vi "UI_(05A)_Set_Record_Start_State.vi"(3 "error in (no error)":errorcluster, 4 "Settings cluster in":T1={"Defaults"={"Default User"=0.0, "VISA Resource Name "="", "Histogram parameters"={"max"=300.0, "min"=0.0, "# bins"=10, "threshold"=8.0, "thr. type"=enum."higher accepted"}}, "Recording and saving"={"Researcher name"="", "Name prefix"="", "Data post-processing"={"Filter type"=enum."Savitzky-Golay", "Length"=31, "Order"=3}, "Stop at"=0.0, "\"Stop at\" enabled"=FALSE, "Default save folder path"=path "", "Acquisition FPS"=enum."Max"}, "Geometry"={"Sensor board size"=enum."", "Bridge swap"=FALSE, "Twisted neck"=FALSE, "Bridge H. offset"=0.0, "Bridge V. offset"=0.0, "Magnets orientation"=0.0, "Cage type"=0, "Cage parameters"={"Round"=variant(i16 0), "Square"=variant(u16 0), "Donut-maze"=variant(u16 0), "T-maze"=variant(u8 0), "Sociability-maze"=variant(u8 0)}}, "IO parameters"={"IO general config."=0, "IO 1 configuration"=0, "IO 2 configuration"=0, "IO 3 configuration"=0, "IO 4 configuration"=0, "Activate ext. RS-232"=0, "IO inversion config."=0, "Sync capability"=1}, "Conditions presets array"=[{"Enabled"=FALSE, "Name"="", "Specifier(s)"=[], "Response"={"Response type"=enum."Air puff", "TTL port"=enum."Port 1", "TTL pulse length, ms"=0.0}, "Has been set"=FALSE}, {"Enabled"=FALSE, "Name"="", "Specifier(s)"=[], "Response"={"Response type"=enum."Air puff", "TTL port"=enum."Port 1", "TTL pulse length, ms"=0.0}, "Has been set"=FALSE}, {"Enabled"=FALSE, "Name"="", "Specifier(s)"=[], "Response"={"Response type"=enum."Air puff", "TTL port"=enum."Port 1", "TTL pulse length, ms"=0.0}, "Has been set"=FALSE}, {"Enabled"=FALSE, "Name"="", "Specifier(s)"=[], "Response"={"Response type"=enum."Air puff", "TTL port"=enum."Port 1", "TTL pulse length, ms"=0.0}, "Has been set"=FALSE}, {"Enabled"=FALSE, "Name"="", "Specifier(s)"=[], "Response"={"Response type"=enum."Air puff", "TTL port"=enum."Port 1", "TTL pulse length, ms"=0.0}, "Has been set"=FALSE}, {"Enabled"=FALSE, "Name"="", "Specifier(s)"=[], "Response"={"Response type"=enum."Air puff", "TTL port"=enum."Port 1", "TTL pulse length, ms"=0.0}, "Has been set"=FALSE}, {"Enabled"=FALSE, "Name"="", "Specifier(s)"=[], "Response"={"Response type"=enum."Air puff", "TTL port"=enum."Port 1", "TTL pulse length, ms"=0.0}, "Has been set"=FALSE}, {"Enabled"=FALSE, "Name"="", "Specifier(s)"=[], "Response"={"Response type"=enum."Air puff", "TTL port"=enum."Port 1", "TTL pulse length, ms"=0.0}, "Has been set"=FALSE}, {"Enabled"=FALSE, "Name"="", "Specifier(s)"=[], "Response"={"Response type"=enum."Air puff", "TTL port"=enum."Port 1", "TTL pulse length, ms"=0.0}, "Has been set"=FALSE}, {"Enabled"=FALSE, "Name"="", "Specifier(s)"=[], "Response"={"Response type"=enum."Air puff", "TTL port"=enum."Port 1", "TTL pulse length, ms"=0.0}, "Has been set"=FALSE}, {"Enabled"=FALSE, "Name"="", "Specifier(s)"=[], "Response"={"Response type"=enum."Air puff", "TTL port"=enum."Port 1", "TTL pulse length, ms"=0.0}, "Has been set"=FALSE}, {"Enabled"=FALSE, "Name"="", "Specifier(s)"=[], "Response"={"Response type"=enum."Air puff", "TTL port"=enum."Port 1", "TTL pulse length, ms"=0.0}, "Has been set"=FALSE}, {"Enabled"=FALSE, "Name"="", "Specifier(s)"=[], "Response"={"Response type"=enum."Air puff", "TTL port"=enum."Port 1", "TTL pulse length, ms"=0.0}, "Has been set"=FALSE}, {"Enabled"=FALSE, "Name"="", "Specifier(s)"=[], "Response"={"Response type"=enum."Air puff", "TTL port"=enum."Port 1", "TTL pulse length, ms"=0.0}, "Has been set"=FALSE}], "Calibration parameters"={"Timing calibration sw/hw"=1.0, "True FPS"=80.0, "True frame time, s"=80.0, "Disp. calibration info"=[]}, "Settings loaded OK"=FALSE} {"Calibration parameters"."True frame time, s" format="%.10g"; "Calibration parameters"."Disp. calibration info"."Speed, µl per ms" format="%.3g"; "Calibration parameters"."True FPS" format="%.10g"; "Calibration parameters"."Timing calibration sw/hw" format="%.10g"; "Conditions presets array"."Specifier(s)"."Validity criteria(s)"."Validity value" min=0.0 step=0.1 format="%.2g"; "Conditions presets array"."Specifier(s)"."Value" step=1.0 format="%#.2g"; "Recording and saving"."Data post-processing"."Order" min=3 max=11 step=2; "Recording and saving"."Data post-processing"."Length" min=5 max=301 step=2; "Geometry"."Cage type" items=["Round", "Square", "Donut-maze", "T-maze", "Sociability maze", ""]}, 5 "All references in":T21) -> (0 "error out":errorcluster, 1 "Settings cluster out":T1={"Defaults"={"Default User"=0.0, "VISA Resource Name "="", "Histogram parameters"={"max"=300.0, "min"=0.0, "# bins"=10, "threshold"=8.0, "thr. type"=enum."higher accepted"}}, "Recording and saving"={"Researcher name"="", "Name prefix"="", "Data post-processing"={"Filter type"=enum."Savitzky-Golay", "Length"=31, "Order"=3}, "Stop at"=0.0, "\"Stop at\" enabled"=FALSE, "Default save folder path"=path "", "Acquisition FPS"=enum."Max"}, "Geometry"={"Sensor board size"=enum."", "Bridge swap"=FALSE, "Twisted neck"=FALSE, "Bridge H. offset"=0.0, "Bridge V. offset"=0.0, "Magnets orientation"=0.0, "Cage type"=0, "Cage parameters"={"Round"=variant(i16 0), "Square"=variant(u16 0), "Donut-maze"=variant(u16 0), "T-maze"=variant(u8 0), "Sociability-maze"=variant(u8 0)}}, "IO parameters"={"IO general config."=0, "IO 1 configuration"=0, "IO 2 configuration"=0, "IO 3 configuration"=0, "IO 4 configuration"=0, "Activate ext. RS-232"=0, "IO inversion config."=0, "Sync capability"=1}, "Conditions presets array"=[{"Enabled"=FALSE, "Name"="", "Specifier(s)"=[], "Response"={"Response type"=enum."Air puff", "TTL port"=enum."Port 1", "TTL pulse length, ms"=0.0}, "Has been set"=FALSE}, {"Enabled"=FALSE, "Name"="", "Specifier(s)"=[], "Response"={"Response type"=enum."Air puff", "TTL port"=enum."Port 1", "TTL pulse length, ms"=0.0}, "Has been set"=FALSE}, {"Enabled"=FALSE, "Name"="", "Specifier(s)"=[], "Response"={"Response type"=enum."Air puff", "TTL port"=enum."Port 1", "TTL pulse length, ms"=0.0}, "Has been set"=FALSE}, {"Enabled"=FALSE, "Name"="", "Specifier(s)"=[], "Response"={"Response type"=enum."Air puff", "TTL port"=enum."Port 1", "TTL pulse length, ms"=0.0}, "Has been set"=FALSE}, {"Enabled"=FALSE, "Name"="", "Specifier(s)"=[], "Response"={"Response type"=enum."Air puff", "TTL port"=enum."Port 1", "TTL pulse length, ms"=0.0}, "Has been set"=FALSE}, {"Enabled"=FALSE, "Name"="", "Specifier(s)"=[], "Response"={"Response type"=enum."Air puff", "TTL port"=enum."Port 1", "TTL pulse length, ms"=0.0}, "Has been set"=FALSE}, {"Enabled"=FALSE, "Name"="", "Specifier(s)"=[], "Response"={"Response type"=enum."Air puff", "TTL port"=enum."Port 1", "TTL pulse length, ms"=0.0}, "Has been set"=FALSE}, {"Enabled"=FALSE, "Name"="", "Specifier(s)"=[], "Response"={"Response type"=enum."Air puff", "TTL port"=enum."Port 1", "TTL pulse length, ms"=0.0}, "Has been set"=FALSE}, {"Enabled"=FALSE, "Name"="", "Specifier(s)"=[], "Response"={"Response type"=enum."Air puff", "TTL port"=enum."Port 1", "TTL pulse length, ms"=0.0}, "Has been set"=FALSE}, {"Enabled"=FALSE, "Name"="", "Specifier(s)"=[], "Response"={"Response type"=enum."Air puff", "TTL port"=enum."Port 1", "TTL pulse length, ms"=0.0}, "Has been set"=FALSE}, {"Enabled"=FALSE, "Name"="", "Specifier(s)"=[], "Response"={"Response type"=enum."Air puff", "TTL port"=enum."Port 1", "TTL pulse length, ms"=0.0}, "Has been set"=FALSE}, {"Enabled"=FALSE, "Name"="", "Specifier(s)"=[], "Response"={"Response type"=enum."Air puff", "TTL port"=enum."Port 1", "TTL pulse length, ms"=0.0}, "Has been set"=FALSE}, {"Enabled"=FALSE, "Name"="", "Specifier(s)"=[], "Response"={"Response type"=enum."Air puff", "TTL port"=enum."Port 1", "TTL pulse length, ms"=0.0}, "Has been set"=FALSE}, {"Enabled"=FALSE, "Name"="", "Specifier(s)"=[], "Response"={"Response type"=enum."Air puff", "TTL port"=enum."Port 1", "TTL pulse length, ms"=0.0}, "Has been set"=FALSE}], "Calibration parameters"={"Timing calibration sw/hw"=1.0, "True FPS"=80.0, "True frame time, s"=80.0, "Disp. calibration info"=[]}, "Settings loaded OK"=FALSE} {"Calibration parameters"."True frame time, s" format="%.10g"; "Calibration parameters"."Disp. calibration info"."Speed, µl per ms" format="%.3g"; "Calibration parameters"."True FPS" format="%.10g"; "Calibration parameters"."Timing calibration sw/hw" format="%.10g"; "Conditions presets array"."Specifier(s)"."Validity criteria(s)"."Validity value" min=0.0 step=0.1 format="%.2g"; "Conditions presets array"."Specifier(s)"."Value" step=1.0 format="%#.2g"; "Recording and saving"."Data post-processing"."Order" min=3 max=11 step=2; "Recording and saving"."Data post-processing"."Length" min=5 max=301 step=2; "Geometry"."Cage type" items=["Round", "Square", "Donut-maze", "T-maze", "Sociability maze", ""]}, 2 "All references out":T21)   [LabVIEW 2018, in "Tracker.lvlib"]
uses:
  Tracker.lvlib
  Controls/CTL_All_References.ctl
  Controls/CTL_Controls_References.ctl
  Controls/CTL_Indicators_References.ctl
  Controls/CTL_Panes_and_VIs_References.ctl
  Controls/CTL_Histogram_Properties.ctl
  <vilib>/Utility/miscctls.llb/LVRangeTypeDef.ctl
  Controls/CTL_Settings_cluster.ctl
  Controls/CTL_Histogram_parameters.ctl
  Controls/CTL_Filter_selector.ctl
  Controls/CTL_Acquisition_speed_selector.ctl
  Controls/CTL_Segmented_plot_parameters_2.ctl
  Libraries/Cage Diagram/Typedefs/CTL_Cage_type.ctl
  Controls/CTL_Cage_all_segmentation_params_set.ctl
  Controls/CTL_IO_params_cluster.ctl
  Controls/CTL_Conditions_Array.ctl
  Controls/CTL_Conditions_Cluster.ctl
  Controls/CTL_Condition_type.ctl
  Controls/CTL_Comparison_type.ctl
  Controls/CTL_Validity_check_criteria.ctl
  Controls/CTL_Response_info.ctl
  Controls/CTL_Condition_response_type.ctl
  Controls/CTL_Reponse_port_info.ctl
  Controls/CTL_Calibration_parameters.ctl
  Controls/CTL_Dispenser_calibration_info.ctl
  <vilib>/Utility/error.llb/Error Cluster From Error Code.vi
  <vilib>/ErrorRing/Error Ring.xnode
  Common_Resources.lvlib
  Libraries/Cage Diagram/Cage Diagram.lvlib
panel:
  in  "Histogram initialization cluster":T19={"X Scale.Range"={"Minimum"=0.0, "Maximum"=13.0, "Increment"=1.0, "Minor Increment"=1.0, "Start"=0.0}, "Caption.Text"="Zone preference (normalized)", "X Scale.Offset and Multiplier:Multiplier"=1.0, "X Scale.Offset and Multiplier:Offset"=0.0, "X Scale.Scale Fit"=2, "X Scale.Display Format:Precision"=0, "Y Scale.Mapping Mode"=0, "Zones preference empty initialized array"=[0, 0, 0, 0, 0, 0, 0, 0, 0, 0, 0, 0, 0, 0], "Plot.Fill/Point Color"=15790320}
  out "Panes references":T24
  out "Controls references params":string[][](array[string])
  out "Indicators references params":string[][](array[string])
  out "Indicators references":T23
  out "Controls references":T22
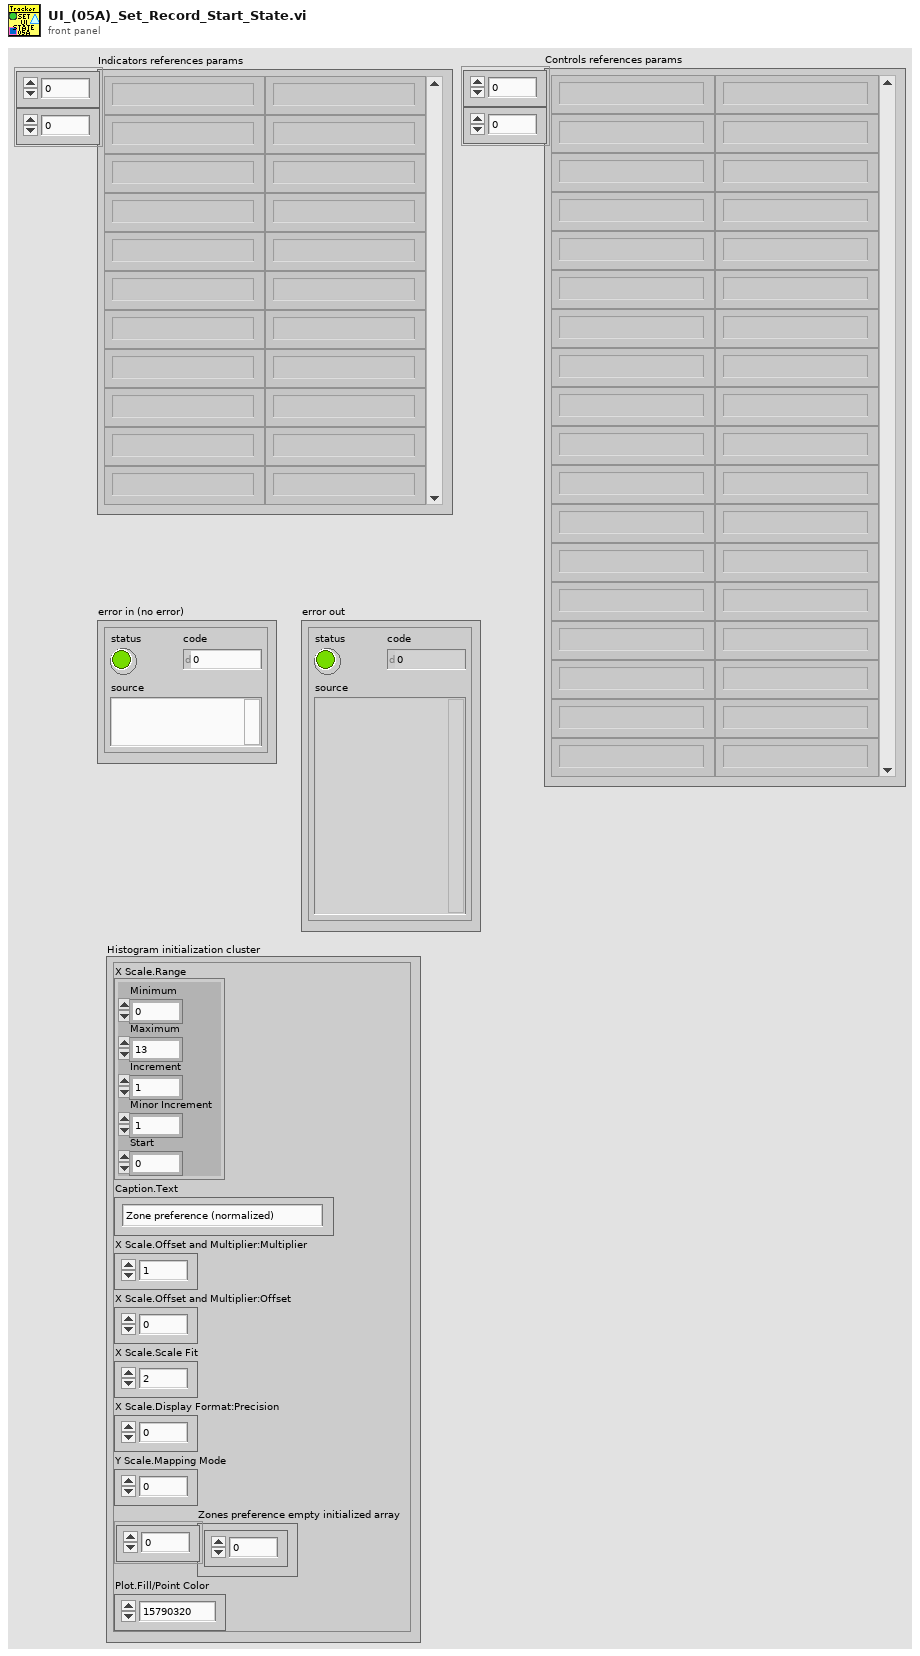
[diagram p1: front panel]
types:
  T1 = typedef "Common_Resources.lvlib/CTL_Settings_cluster.ctl" = cluster{"Defaults":cluster{"Default User":dbl, "VISA Resource Name ":string, "Histogram parameters":T2}, "Recording and saving":cluster{"Researcher name":string, "Name prefix":string, "Data post-processing":T3, "Stop at":dbl, "\"Stop at\" enabled":bool, "Default save folder path":path, "Acquisition FPS":T4}, "Geometry":T5, "IO parameters":T8, "Conditions presets array":T9, "Calibration parameters":T17, "Settings loaded OK":bool}
  T2 = typedef "Common_Resources.lvlib/CTL_Histogram_parameters.ctl" = cluster{"max":dbl, "min":dbl, "# bins":i32, "threshold":dbl, "thr. type":enum16{"higher accepted", "lower accepted"}}
  T3 = typedef "Common_Resources.lvlib/CTL_Filter_selector.ctl" = cluster{"Filter type":enum16{"None", "Savitzky-Golay"}, "Length":i32, "Order":i32}
  T4 = typedef "Common_Resources.lvlib/CTL_Acquisition_speed_selector.ctl" = enum16{"Max", "Optimal", "Eco"}
  T5 = typedef "Common_Resources.lvlib/CTL_Segmented_plot_parameters_2.ctl" = cluster{"Sensor board size":enum16{"", "Large"}, "Bridge swap":bool, "Twisted neck":bool, "Bridge H. offset":sgl, "Bridge V. offset":sgl, "Magnets orientation":sgl, "Cage type":T6, "Cage parameters":T7}
  T6 = typedef "Cage Diagram.lvlib/CTL_Cage_type.ctl" = u16
  T7 = typedef "Common_Resources.lvlib/CTL_Cage_all_segmentation_params_set.ctl" = cluster{"Round":variant, "Square":variant, "Donut-maze":variant, "T-maze":variant, "Sociability-maze":variant}
  T8 = typedef "Common_Resources.lvlib/CTL_IO_params_cluster.ctl" = cluster{"IO general config.":u16, "IO 1 configuration":u16, "IO 2 configuration":u16, "IO 3 configuration":u16, "IO 4 configuration":u16, "Activate ext. RS-232":u16, "IO inversion config.":u16, "Sync capability":u8}
  T9 = typedef "Common_Resources.lvlib/CTL_Conditions_Array.ctl" = T10[]
  T10 = typedef "Common_Resources.lvlib/CTL_Conditions_Cluster.ctl" = cluster{"Enabled":bool, "Name":string, "Specifier(s)":cluster{"Specifier enabled":bool, "Condition type":T11, "Comparison type":T12, "Value":dbl, "Validity criteria(s)":cluster{"V. check enabled":bool, "Criteria":T13, "Validity value":dbl}[]}[], "Response":T14, "Has been set":bool}
  T11 = typedef "Common_Resources.lvlib/CTL_Condition_type.ctl" = enum16{"Speed", "Zone", "Angle to wall"}
  T12 = typedef "Common_Resources.lvlib/CTL_Comparison_type.ctl" = enum16{"Less", "Less or Equal", "Equal", "Greater or Equal", "Greater", "Not Equal"}
  T13 = typedef "Common_Resources.lvlib/CTL_Validity_check_criteria.ctl" = enum16{"Running bout (seconds)", "Running bout (meters)"}
  T14 = typedef "Common_Resources.lvlib/CTL_Response_info.ctl" = cluster{"Response type":T15, "TTL port":T16, "TTL pulse length, ms":dbl}
  T15 = typedef "Common_Resources.lvlib/CTL_Condition_response_type.ctl" = enum16{"None", "Air puff", "Liquid reward", "TTL pulse", "TTL pulse (ubr)", "TTL signal"}
  T16 = typedef "Common_Resources.lvlib/CTL_Reponse_port_info.ctl" = enum16{"Port 1", "Port 2", "Port 3", "Port 4"}
  T17 = typedef "Common_Resources.lvlib/CTL_Calibration_parameters.ctl" = cluster{"Timing calibration sw/hw":dbl, "True FPS":dbl, "True frame time, s":dbl, "Disp. calibration info":T18}
  T18 = typedef "Common_Resources.lvlib/CTL_Dispenser_calibration_info.ctl" = cluster{"Channel":u8, "Speed, µl per ms":dbl}[]
  T19 = typedef "Common_Resources.lvlib/CTL_Histogram_Properties.ctl" = cluster{"X Scale.Range":T20, "Caption.Text":string, "X Scale.Offset and Multiplier:Multiplier":dbl, "X Scale.Offset and Multiplier:Offset":dbl, "X Scale.Scale Fit":u8, "X Scale.Display Format:Precision":u8, "Y Scale.Mapping Mode":u8, "Zones preference empty initialized array":i32[], "Plot.Fill/Point Color":u32}
  T20 = typedef "LVRangeTypeDef.ctl" = cluster{"Minimum":dbl, "Maximum":dbl, "Increment":dbl, "Minor Increment":dbl, "Start":dbl}
  T21 = typedef "Common_Resources.lvlib/CTL_All_References.ctl" = cluster{"Controls references":T22, "Indicators references":T23, "Service references":T24}
  T22 = typedef "Common_Resources.lvlib/CTL_Controls_References.ctl" = cluster{"Check HW connection":refnum<vi>, "Save settings":refnum<vi>, "Reset zones":refnum<vi>, "Reset stimuli":refnum<vi>, "Record/Stop":refnum<vi>, "Reset barplot":refnum<vi>, "Multiplyer of chart RX":refnum<vi>, "Show zones":refnum<vi>, "Show magnets":refnum<vi>, "Show heatmap":refnum<vi>, "Show full track":refnum<vi>, "Open File":refnum<vi>, "Play/Pause":refnum<vi>, "Trace, s":refnum<vi>, "Playback speed":refnum<vi>, "Timeline":refnum<vi>, "By Zone stim. setup":refnum<vi>, "Set/Rec and Analyse Tab":refnum<vi>, "Cage radial segmentation":refnum<vi>, "Set IO config":refnum<vi>, "Rainbow (time)":refnum<vi>, "Rainbow (speed)":refnum<vi>, "Add Reward":refnum<vi>, "Modify Reward":refnum<vi>, "Delete Reward":refnum<vi>, "Speed threshold, mm/s":refnum<vi>, "Start Over":refnum<vi>}
  T23 = typedef "Common_Resources.lvlib/CTL_Indicators_References.ctl" = cluster{"HW info":refnum<vi>, "Port":refnum<vi>, "Ready":refnum<vi>, "IO status indicator":refnum<vi>, "Current Time":refnum<vi>, "Record timestamp":refnum<vi>, "Mouse speed":refnum<vi>, "Mouse speed, mm/s":refnum<vi>, "Running, perc. of time":refnum<vi>, "Histograms":refnum<vi>, "Cage size":refnum<vi>, "Reward":refnum<vi>, "Current zone":refnum<vi>, "Run length, m":refnum<vi>}
  T24 = typedef "Common_Resources.lvlib/CTL_Panes_and_VIs_References.ctl" = cluster{"Pane":refnum<vi>, "This VI":refnum<vi>, "Menu":refnum<k9>}
  T25 = enum8{"Enabled", "Disabled", "Disabled and Grayed Out"}
  T26 = cluster{"Slider":dbl, "Slider":dbl, "Slider":dbl}
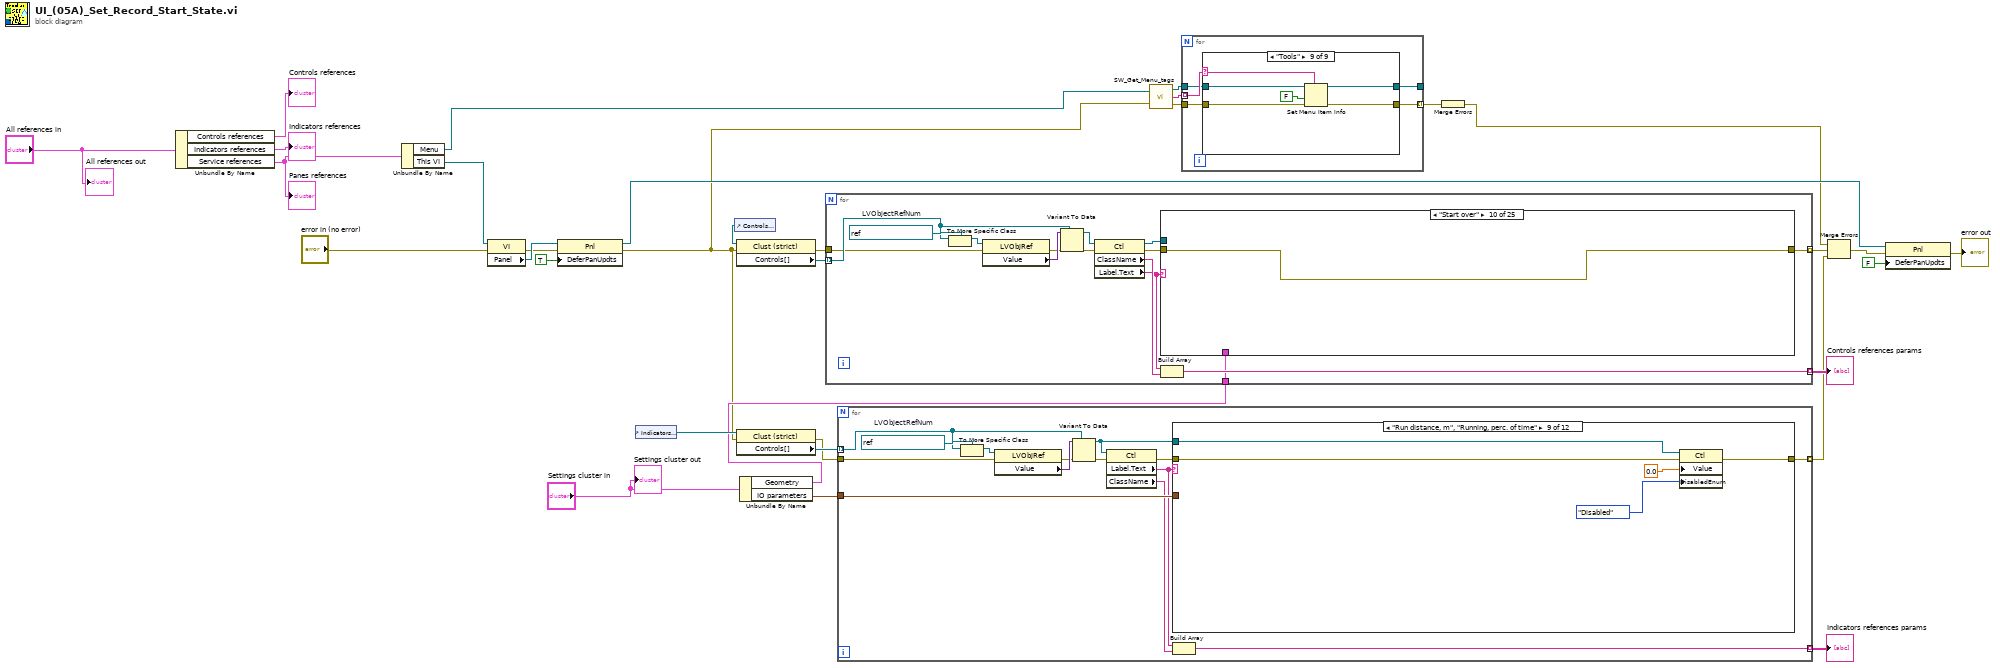
[diagram p0: block diagram]
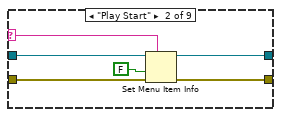
[diagram p3: hidden frame]
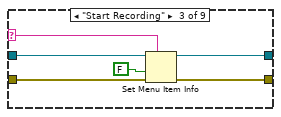
[diagram p4: hidden frame]
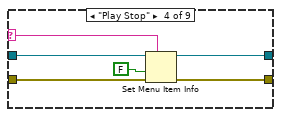
[diagram p5: hidden frame]
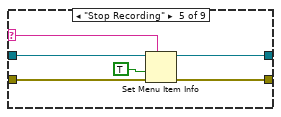
[diagram p6: hidden frame]
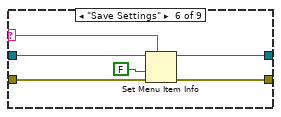
[diagram p7: hidden frame]
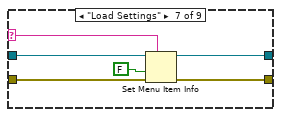
[diagram p8: hidden frame]
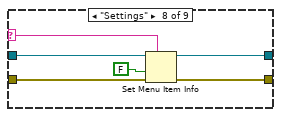
[diagram p9: hidden frame]
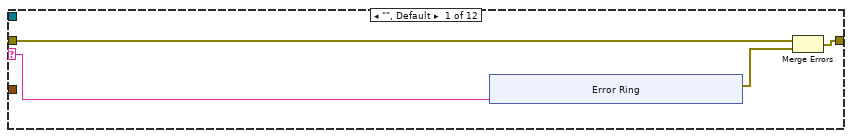
[diagram p10: hidden frame]
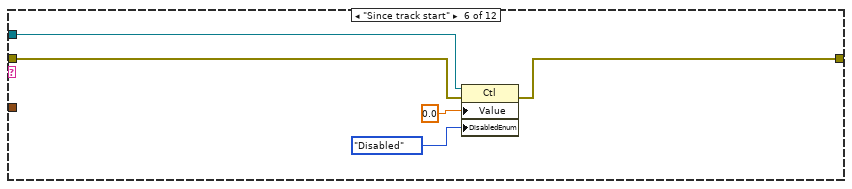
[diagram p15: hidden frame]
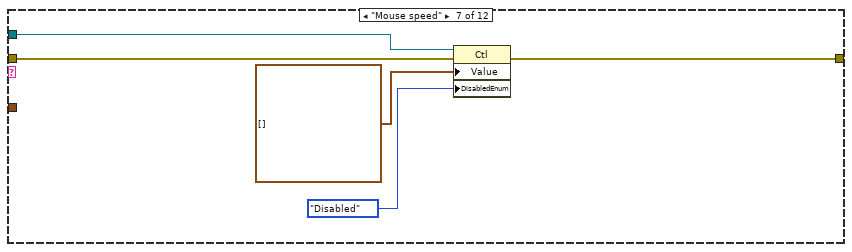
[diagram p16: hidden frame]
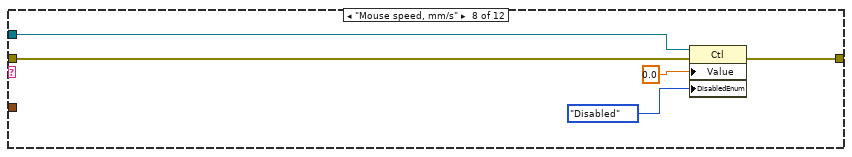
[diagram p17: hidden frame]
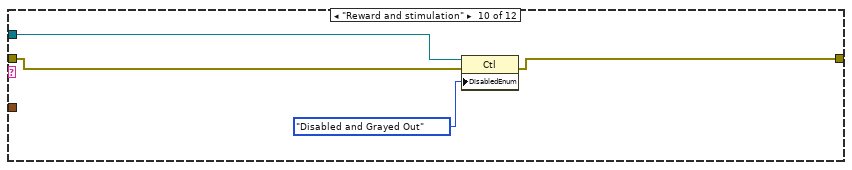
[diagram p18: hidden frame]
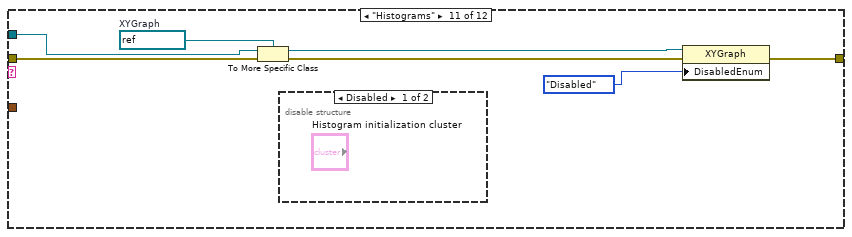
[diagram p19: hidden frame]
diagram:
  n1 = Unbundle By Name("All references in") -> ("Controls references"=→"Controls references":T22, "Indicators references"=→"Indicators references":T23, "Service references"=w24:T24)
  "Panes references" <- w24
  n2 = Unbundle By Name(w24) -> ("Menu"=w3:refnum<k9>, "This VI"=w21:refnum<vi>)
  n3 = property class="VI"(reference=w21, error in="error in (no error)") -> (error out=w14:errorcluster, "Panel"=w23:refnum<vi>)  [unwired: 1 out]
  n4 = property class="Pnl"(reference=w23, error in=w14, "DeferPanUpdts"=TRUE ("Defer Panel Updates")) -> (reference out=w15:refnum<vi>, error out=w2:errorcluster)
  n5 = control-ref of="Indicators references"() -> (w27:refnum<vi>)
  n6 = control-ref of="Controls references"() -> (w29:refnum<vi>)
  n7 = property class="Clust (strict)"(reference=w29, error in=w2) -> (error out=w20:errorcluster, "Controls[]"=w30:refnum<vi>[])  [unwired: 1 out]
  n8 = property class="Clust (strict)"(reference=w27, error in=w2) -> (error out=w19:errorcluster, "Controls[]"=w28:refnum<vi>[])  [unwired: 1 out]
  n9 = Unbundle By Name("Settings cluster in") -> ("Geometry"=w8:T5, "IO parameters"=w10:T8)
  n10 = for {
    tunnel: w30 -> [w45] mode=indexing
    tunnel: [w42] -> w25 mode=indexing
    tunnel: w20 -> [w41]
    tunnel: [w37] -> w12 mode=indexing
    tunnel: w8 -> [w34]
    w47 = refnum<vi> refnum  # LVObjectRefNum
    n11 = To More Specific Class(target class=w47, reference=w45) -> (specific class reference=w48:refnum<vi>)  [unwired: 1 in, 1 out]
    n12 = property class="LVObjRef"(reference=w48, error in=w41) -> (error out=w40:errorcluster, "Value"=w46:variant)  [unwired: 1 out]
    n13 = Variant To Data(error in=w40, type=w45, Variant=w46) -> (data=w44:refnum<vi>, error out=w39:errorcluster)
    n14 = property class="Ctl"(reference=w44, error in=w39) -> (reference out=w35:refnum<vi>, error out=w36:errorcluster, "ClassName"=w43:string, "Label.Text"=w38:string)
    n15 = case shown="\"Start over\"" w38 {
      selector: w38 -> [w49 _ _ _ _ _ _ _ _ _ _ _ _ _ _ _ _ _ _ _ _ _ _ _ _]
      tunnel: [w51 w62 w67 w74 w75 w76 w77 w78 w80 w87 w90 w98 w106 w112 w113 w120 w130 w138 w144 w145 w154 w161 w169 w182 w188] -> w37
      tunnel: w36 -> [w52 w66 w69 w74 w75 w76 w77 w78 w81 w87 w92 w100 w108 w112 w115 w122 w132 w140 w144 w146 w156 w163 w171 w184 w188]
      tunnel: w35 -> [_ w65 w68 _ _ _ _ _ w82 _ w95 w103 w111 _ w114 w121 w135 w143 _ w147 w159 w166 w174 w187 _]
      tunnel: w34 -> [_ _ _ _ _ _ _ _ _ _ _ _ _ _ _ _ _ _ _ _ _ _ _ _ _]
      frame "", Default {
        n16 = xnode "Error Ring"("parameter 0"=w49) -> ("error out"=w50:errorcluster)
        n17 = Merge Errors(w52, w50) -> (w51:errorcluster)
      }
      frame "Cage radial segmentation" {
        w64 = refnum<vi> refnum  # Cluster
        n18 = To More Specific Class(target class=w64, reference=w65, error in=w66) -> (specific class reference=w61:refnum<vi>, error out=w63:errorcluster)
        n19 = property class="Clust"(reference=w61, error in=w63, "DisabledEnum"=T25."Disabled and Grayed Out" ("Disabled")) -> (error out=w62:errorcluster)  [unwired: 1 out]
      }
      frame "Set/Rec and Analyse Tab" {
        w73 = refnum<vi> refnum  # TabControl
        n20 = To More Specific Class(target class=w73, reference=w68, error in=w69) -> (specific class reference=w71:refnum<vi>, error out=w72:errorcluster)
        n21 = property class="TabCtl"(reference=w71, error in=w72, "Value"=enum32{"Settings", "Recording and Analysis"}."Recording and Analysis" ("Set/Rec and Analyse Tab")) -> (error out=w67:errorcluster)  [unwired: 1 out]
      }
      frame "Check HW connection" {
      }
      frame "Save settings" {
      }
      frame "Set IO config" {
      }
      frame "Reset zones" {
      }
      frame "Reset stimuli" {
      }
      frame "Record/Stop" {
        w83 = refnum<vi> refnum  # Boolean
        n22 = To More Specific Class(target class=w83, reference=w82, error in=w81) -> (specific class reference=w86:refnum<vi>, error out=w85:errorcluster)
        n23 = property class="Bool"(reference=w86, error in=w85, "DisabledEnum"=T25."Enabled" ("Disabled"), "Value"=TRUE) -> (error out=w80:errorcluster)  [unwired: 1 out]
      }
      frame "Start over" {
      }
      frame "Reset barplot" {
        w94 = refnum<vi> refnum  # Boolean
        n24 = To More Specific Class(target class=w94, reference=w95, error in=w92) -> (specific class reference=w93:refnum<vi>, error out=w91:errorcluster)
        n25 = property class="Bool"(reference=w93, error in=w91, "Value"=FALSE, "DisabledEnum"=T25."Enabled" ("Disabled")) -> (error out=w90:errorcluster)  [unwired: 1 out]
      }
      frame "Multiplyer of chart RX" {
        w102 = refnum<vi> refnum  # Slide
        n26 = To More Specific Class(target class=w102, reference=w103, error in=w100) -> (specific class reference=w101:refnum<vi>, error out=w99:errorcluster)
        n27 = property class="Slide"(reference=w101, error in=w99, "Value"=u8 1, "DisabledEnum"=T25."Enabled" ("Disabled")) -> (error out=w98:errorcluster)  [unwired: 1 out]
      }
      frame "Show zones" {
        w110 = refnum<vi> refnum  # Boolean
        n28 = To More Specific Class(target class=w110, reference=w111, error in=w108) -> (specific class reference=w109:refnum<vi>, error out=w107:errorcluster)
        n29 = property class="Bool"(reference=w109, error in=w107, "Value"=TRUE, "DisabledEnum"=T25."Enabled" ("Disabled")) -> (error out=w106:errorcluster)  [unwired: 1 out]
      }
      frame "Show magnets" {
      }
      frame "Rainbow (speed)", "Rainbow (time)" {
        w116 = refnum<vi> refnum  # Boolean
        n30 = To More Specific Class(target class=w116, reference=w114, error in=w115) -> (specific class reference=w118:refnum<vi>, error out=w119:errorcluster)
        n31 = property class="Bool"(reference=w118, error in=w119, "DisabledEnum"=T25."Enabled" ("Disabled")) -> (error out=w113:errorcluster)  [unwired: 1 out]
      }
      frame "Add Reward", "Modify Reward", "Remove Reward" {
        w127 = refnum<vi> refnum  # Boolean
        n32 = To More Specific Class(target class=w127, reference=w121, error in=w122) -> (specific class reference=w126:refnum<vi>, error out=w125:errorcluster)
        n33 = property class="Bool"(reference=w126, error in=w125, "Value"=FALSE, "DisabledEnum"=T25."Disabled and Grayed Out" ("Disabled")) -> (error out=w120:errorcluster)  [unwired: 1 out]
      }
      frame "Show heatmap" {
        w134 = refnum<vi> refnum  # Boolean
        n34 = To More Specific Class(target class=w134, reference=w135, error in=w132) -> (specific class reference=w133:refnum<vi>, error out=w131:errorcluster)
        n35 = property class="Bool"(reference=w133, error in=w131, "Value"=FALSE, "DisabledEnum"=T25."Disabled and Grayed Out" ("Disabled")) -> (error out=w130:errorcluster)  [unwired: 1 out]
      }
      frame "Show full track" {
        w142 = refnum<vi> refnum  # Boolean
        n36 = To More Specific Class(target class=w142, reference=w143, error in=w140) -> (specific class reference=w141:refnum<vi>, error out=w139:errorcluster)
        n37 = property class="Bool"(reference=w141, error in=w139, "Value"=FALSE, "DisabledEnum"=T25."Disabled and Grayed Out" ("Disabled")) -> (error out=w138:errorcluster)  [unwired: 1 out]
      }
      frame "Open File" {
      }
      frame "Play/Pause" {
        w148 = refnum<vi> refnum  # Boolean
        n38 = To More Specific Class(target class=w148, reference=w147, error in=w146) -> (specific class reference=w151:refnum<vi>, error out=w150:errorcluster)
        n39 = property class="Bool"(reference=w151, error in=w150, "DisabledEnum"=T25."Disabled and Grayed Out" ("Disabled")) -> (error out=w145:errorcluster)  [unwired: 1 out]
      }
      frame "Trace, s" {
        w158 = refnum<vi> refnum  # Slide
        n40 = To More Specific Class(target class=w158, reference=w159, error in=w156) -> (specific class reference=w157:refnum<vi>, error out=w155:errorcluster)
        n41 = property class="Slide"(reference=w157, error in=w155, "Value"=u8 5, "DisabledEnum"=T25."Enabled" ("Disabled")) -> (error out=w154:errorcluster)  [unwired: 1 out]
      }
      frame "Speed threshold" {
        w165 = refnum<vi> refnum  # Digital
        n42 = To More Specific Class(target class=w165, reference=w166, error in=w163) -> (specific class reference=w164:refnum<vi>, error out=w162:errorcluster)
        n43 = property class="DigNum"(reference=w164, error in=w162, "DisabledEnum"=T25."Enabled" ("Disabled")) -> (error out=w161:errorcluster)  [unwired: 1 out]
      }
      frame "Playback speed" {
        w173 = refnum<vi> refnum  # Ring
        n44 = To More Specific Class(target class=w173, reference=w174, error in=w171) -> (specific class reference=w172:refnum<vi>, error out=w170:errorcluster)
        n45 = property class="Ring"(reference=w172, error in=w170, "Value"=u8 3, "DisabledEnum"=T25."Disabled and Grayed Out" ("Disabled")) -> (error out=w169:errorcluster)  [unwired: 1 out]
      }
      frame "Timeline" {
        w176 = 0.0 ("Slider")
        w186 = refnum<vi> refnum  # Slide
        n46 = To More Specific Class(target class=w186, reference=w187, error in=w184) -> (specific class reference=w185:refnum<vi>, error out=w183:errorcluster)
        n47 = Bundle(cluster=T26 {"Slider"=0.0, "Slider"=0.0, "Slider"=0.0} ("Timeline"), "Slider"=w176, "Slider"=0.001, "Slider"=w176) -> (w179:T26)
        n48 = To Variant(anything=w179) -> (Variant=w178:variant)
        n49 = property class="Slide"(reference=w185, error in=w183, "Value"=w178, "DisabledEnum"=T25."Disabled" ("Disabled"), "Scale.Maximum"=60.0 ("Scale.Range:Maximum")) -> (error out=w182:errorcluster)  [unwired: 1 out]
      }
      frame "By Zone stim. setup" {
      }
    }
    n50 = Build Array(w38, w43) -> (w42:string[])
  }
  "Controls references params" <- w25
  n51 = for {
    tunnel: w28 -> [w199] mode=indexing
    tunnel: [w189] -> w26 mode=indexing
    tunnel: w19 -> [w197]
    tunnel: [w193] -> w18 mode=indexing
    tunnel: w10 -> [w192]
    w201 = refnum<vi> refnum  # LVObjectRefNum
    n52 = To More Specific Class(target class=w201, reference=w199) -> (specific class reference=w202:refnum<vi>)  [unwired: 1 in, 1 out]
    n53 = property class="LVObjRef"(reference=w202, error in=w197) -> (error out=w196:errorcluster, "Value"=w200:variant)  [unwired: 1 out]
    n54 = Variant To Data(error in=w196, type=w199, Variant=w200) -> (data=w198:refnum<vi>, error out=w195:errorcluster)
    n55 = property class="Ctl"(reference=w198, error in=w195) -> (error out=w194:errorcluster, "Label.Text"=w191:string, "ClassName"=w190:string)  [unwired: 1 out]
    n56 = case shown="\"Run distance, m\", \"Running, perc. of time\"" w191 {
      selector: w191 -> [w203 _ _ _ _ _ _ _ _ _ _ _]
      tunnel: w198 -> [_ _ _ _ _ w218 w227 w232 w237 w238 w248 _]
      tunnel: w194 -> [w206 w214 w215 w216 w217 w220 w226 w231 w236 w240 w244 w249]
      tunnel: [w205 w214 w215 w216 w217 w219 w225 w230 w235 w239 w247 w249] -> w193
      tunnel: w192 -> [_ _ _ _ _ _ _ _ _ _ _ _]
      frame "", Default {
        n57 = xnode "Error Ring"("parameter 0"=w203) -> ("error out"=w204:errorcluster)
        n58 = Merge Errors(w206, w204) -> (w205:errorcluster)
      }
      frame "Cage size", "HW info", "Port" {
      }
      frame "Ready" {
      }
      frame "IO status indicator" {
      }
      frame "Current Time" {
      }
      frame "Since track start" {
        n59 = property class="Ctl"(reference=w218, error in=w220, "Value"=0.0, "DisabledEnum"=T25."Disabled" ("Disabled")) -> (error out=w219:errorcluster)  [unwired: 1 out]
      }
      frame "Mouse speed" {
        n60 = property class="Ctl"(reference=w227, error in=w226, "Value"=waveform(dbl)[] [] ("History Data"), "DisabledEnum"=T25."Disabled" ("Disabled")) -> (error out=w225:errorcluster)  [unwired: 1 out]
      }
      frame "Mouse speed, mm/s" {
        n61 = property class="Ctl"(reference=w232, error in=w231, "Value"=0.0, "DisabledEnum"=T25."Disabled" ("Disabled")) -> (error out=w230:errorcluster)  [unwired: 1 out]
      }
      frame "Run distance, m", "Running, perc. of time" {
        n62 = property class="Ctl"(reference=w237, error in=w236, "Value"=0.0, "DisabledEnum"=T25."Disabled" ("Disabled")) -> (error out=w235:errorcluster)  [unwired: 1 out]
      }
      frame "Reward and stimulation" {
        n63 = property class="Ctl"(reference=w238, error in=w240, "DisabledEnum"=T25."Disabled and Grayed Out" ("Disabled")) -> (error out=w239:errorcluster)  [unwired: 1 out]
      }
      frame "Histograms" {
        w245 = refnum<vi> refnum  # XYGraph
        n64 = To More Specific Class(target class=w245, reference=w248, error in=w244) -> (specific class reference=w246:refnum<vi>, error out=w243:errorcluster)
        n65 = disable-structure shown="Disabled" {
          frame Disabled {
          }
          frame Enabled {
          }
        }
        n66 = property class="XYGraph"(reference=w246, error in=w243, "DisabledEnum"=T25."Disabled" ("Disabled")) -> (error out=w247:errorcluster)  [unwired: 1 out]
      }
      frame "Current zone" {
      }
    }
    n67 = Build Array(w191, w190) -> (w189:string[])
  }
  "Indicators references params" <- w26
  n68 = call "SW_Get_Menu_tags.vi"("Menu ref in"=w3, "error in (no error)"=w2) -> ("Menu ref out"=w5:refnum<k9>, "(Sub)menu tags"=w7:string[], "error out"=w6:errorcluster)
  n69 = for {
    tunnel: w7 -> [w254] mode=indexing
    tunnel: w6 -> [w253]
    tunnel: [w252] -> w4 mode=indexing
    tunnel: [w251] -> _
    tunnel: w5 -> [w250]
    n70 = case shown="\"Tools\"" w254 {
      selector: w254 -> [_ w262 w268 w274 w280 w286 w292 w298 w304]
      tunnel: w253 -> [w256 w260 w266 w272 w278 w284 w290 w296 w302]
      tunnel: [w256 w259 w265 w271 w277 w283 w289 w295 w301] -> w252
      tunnel: [w255 w258 w264 w270 w276 w282 w288 w294 w300] -> w251
      tunnel: w250 -> [w255 w257 w263 w269 w275 w281 w287 w293 w299]
      frame "", Default {
      }
      frame "Play Start" {
        n71 = Set Menu Item Info(7:w262, 8:w260, 9:FALSE ("enabled"), 11:w257) -> (0:w259:errorcluster, 3:w258:refnum<k9>)  [unwired: 3 in]
      }
      frame "Start Recording" {
        n72 = Set Menu Item Info(7:w268, 8:w266, 9:FALSE ("enabled"), 11:w263) -> (0:w265:errorcluster, 3:w264:refnum<k9>)  [unwired: 3 in]
      }
      frame "Play Stop" {
        n73 = Set Menu Item Info(7:w274, 8:w272, 9:FALSE ("enabled"), 11:w269) -> (0:w271:errorcluster, 3:w270:refnum<k9>)  [unwired: 3 in]
      }
      frame "Stop Recording" {
        n74 = Set Menu Item Info(7:w280, 8:w278, 9:TRUE ("enabled"), 11:w275) -> (0:w277:errorcluster, 3:w276:refnum<k9>)  [unwired: 3 in]
      }
      frame "Save Settings" {
        n75 = Set Menu Item Info(7:w286, 8:w284, 9:FALSE ("enabled"), 11:w281) -> (0:w283:errorcluster, 3:w282:refnum<k9>)  [unwired: 3 in]
      }
      frame "Load Settings" {
        n76 = Set Menu Item Info(7:w292, 8:w290, 9:FALSE ("enabled"), 11:w287) -> (0:w289:errorcluster, 3:w288:refnum<k9>)  [unwired: 3 in]
      }
      frame "Settings" {
        n77 = Set Menu Item Info(7:w298, 8:w296, 9:FALSE ("enabled"), 11:w293) -> (0:w295:errorcluster, 3:w294:refnum<k9>)  [unwired: 3 in]
      }
      frame "Tools" {
        n78 = Set Menu Item Info(7:w304, 8:w302, 9:FALSE ("enabled"), 11:w299) -> (0:w301:errorcluster, 3:w300:refnum<k9>)  [unwired: 3 in]
      }
    }
  }
  n79 = Merge Errors(w4) -> (w1:errorcluster)
  n80 = Merge Errors(w1, w12, w18) -> (w17:errorcluster)
  n81 = property class="Pnl"(reference=w15, error in=w17, "DeferPanUpdts"=FALSE ("Defer Panel Updates")) -> (error out=→"error out":errorcluster)  [unwired: 1 out]
  "All references out" <- "All references in"
  "Settings cluster out" <- "Settings cluster in"
